vi "Destroy All DAQmx Refs.vi"(8 "error in (no error)":errorcluster, 11 "DAQ":refnum<class "DAQ.lvclass">) -> (0 "error out":errorcluster, 3 "DAQ":refnum<class "DAQ.lvclass">)   [LabVIEW 2017, in "DAQ.lvclass"]
doc: "Developed by Kevin Thompson\nkevin@thompsonengineering.net\n\nCopyright 2018-2020\nThompson Engineering, LLC"
uses:
  DAQ.lvclass
  DAQ.lvclass/DAQ.ctl
  DataTypes/TD AO Channel--cluster.ctl
  DataTypes/TD DataValueConversion--cluster.ctl
  DataTypes/TD DO Channel--cluster.ctl
  Accessors/Get DAQNodes Dict.vi
  Accessors/Get DO IONames.vi
  Accessors/Get AO IONames.vi
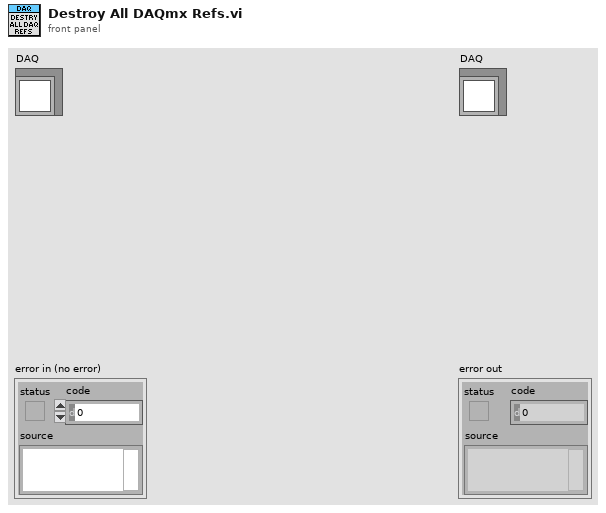
[diagram p1: front panel]
types:
  T1 = typedef "TD Dynamic CVT DVR--ref.ctl" = refnum<data-value>
  T2 = typedef "DAQ.lvclass/TD AO Channel--cluster.ctl" = cluster{"DevName":string, "IOName":string, "IOPath":string, "SchemName":string, "Vmin":dbl, "Vmax":dbl, "Conversion":T3, "DAQmx Task":refnum<k21>}
  T3 = typedef "DAQ.lvclass/TD DataValueConversion--cluster.ctl" = cluster{"MaxSignal":dbl, "MinSignal":dbl, "MaxEngUnit":dbl, "MinEngUnit":dbl, "ScaleOffset":dbl, "negate":bool}
  T4 = typedef "DAQ.lvclass/TD DO Channel--cluster.ctl" = cluster{"DevName":string, "IOName":string, "IOPath":string, "SchemName":string, "logic":enum16{"Lo", "Hi"}, "DAQmx Task":refnum<k21>}
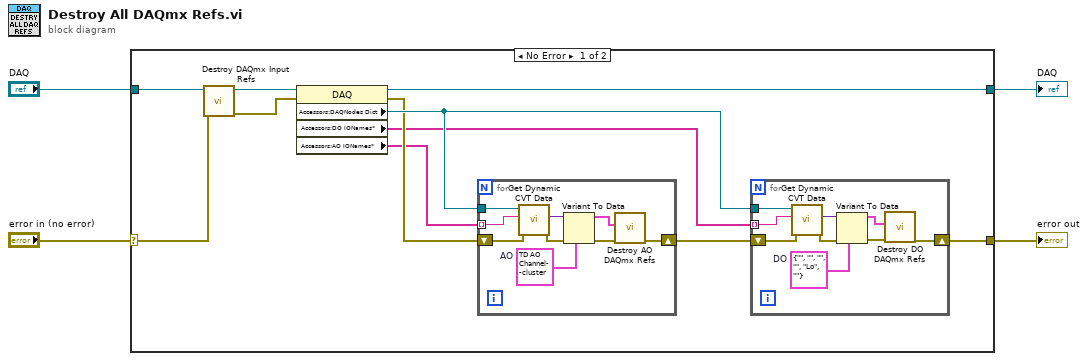
[diagram p0: block diagram]
diagram:
  n1 = case shown="No Error" "error in (no error)" {
    selector: "error in (no error)" -> [w14 w35]
    tunnel: [w13 w35] -> w3
    tunnel: [w11 w34] -> w1
    tunnel: "DAQ" -> [w15 w34]
    frame No Error {
      n2 = call "Destroy DAQmx Input Refs.vi"("error in (no error)"=w14, "DAQ"=w15) -> ("error out"=w8:errorcluster, "DAQ"=w12:refnum<class "DAQ.lvclass">)  [unwired: 8 in]
      n3 = property class="DAQ"(reference=w12, error in=w8) -> (reference out=w11:refnum<class "DAQ.lvclass">, error out=w7:errorcluster, "Accessors:DAQNodes Dict"=w10:T1, "Accessors:DO IONames*"=w6:string[], "Accessors:AO IONames*"=w5:string[])
      n4 = for {
        tunnel: w10 -> [w33]
        tunnel: w5 -> [w32] mode=indexing
        shift-right: [w25] -> w9
        shift-left: w7 -> [w29]
        w27 = T2 {"DevName"="", "IOName"="", "IOPath"="", "SchemName"="", "Vmin"=0.0, "Vmax"=0.0, "Conversion"={"MaxSignal"=0.0, "MinSignal"=0.0, "MaxEngUnit"=0.0, "MinEngUnit"=0.0, "ScaleOffset"=0.0, "negate"=FALSE}, "DAQmx Task"=""}  # AO
        n5 = call <vilib>:"Get Dynamic CVT Data.vi"("error in (no error)"=w29, "DataName"=w32, "dCVT DVR"=w33) -> ("error out"=w30:errorcluster, "value"=w31:variant)  [unwired: 5 in, 2 out]
        n6 = Variant To Data(error in=w30, type=w27, Variant=w31) -> (data=w26:T2, error out=w28:errorcluster)
        n7 = call "Destroy AO DAQmx Refs.vi"("error in (no error)"=w28, "AO"=w26) -> ("error out"=w25:errorcluster)  [unwired: 8 in, 1 out]
      }
      n8 = for {
        tunnel: w10 -> [w24]
        tunnel: w6 -> [w23] mode=indexing
        shift-right: [w16] -> w13
        shift-left: w9 -> [w20]
        w19 = T4 {"DevName"="", "IOName"="", "IOPath"="", "SchemName"="", "logic"=enum."Lo", "DAQmx Task"=""}  # DO
        n9 = call <vilib>:"Get Dynamic CVT Data.vi"("error in (no error)"=w20, "DataName"=w23, "dCVT DVR"=w24) -> ("error out"=w21:errorcluster, "value"=w22:variant)  [unwired: 5 in, 2 out]
        n10 = Variant To Data(error in=w21, type=w19, Variant=w22) -> (data=w18:T4, error out=w17:errorcluster)
        n11 = call "Destroy DO DAQmx Refs.vi"("error in (no error)"=w17, "DO"=w18) -> ("error out"=w16:errorcluster)  [unwired: 8 in, 1 out]
      }
    }
    frame Error {
    }
  }
  "error out" <- w3
  "DAQ" <- w1
